vi "New Line from Strings.vi"(0 "Time":string, 1 "Date":string, 2 "Time Stamp":string, 5 "RunName":string, 6 "DAQ Potential (milliVolts)":string, 7 "Delimiter Character":string, 8 "DAQ Resistance (Ohms)":string, 9 "Mode":string, 10 "DAQ Temperature (deg Celsius)":string, 11 "Setting":string, 12 "BK V":string, 13 "BK C":string, 14 "BK R":string, 15 "BK W":string) -> (4 "Line Produced":string)   [LabVIEW 2010]
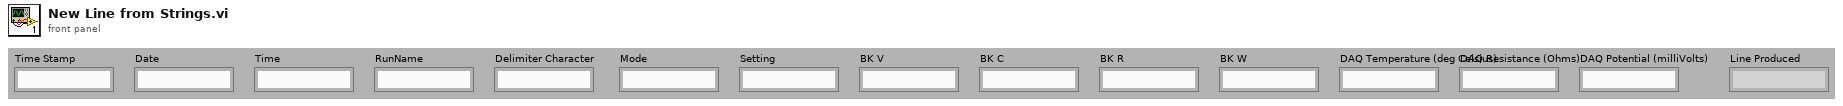
[diagram p1: front panel]
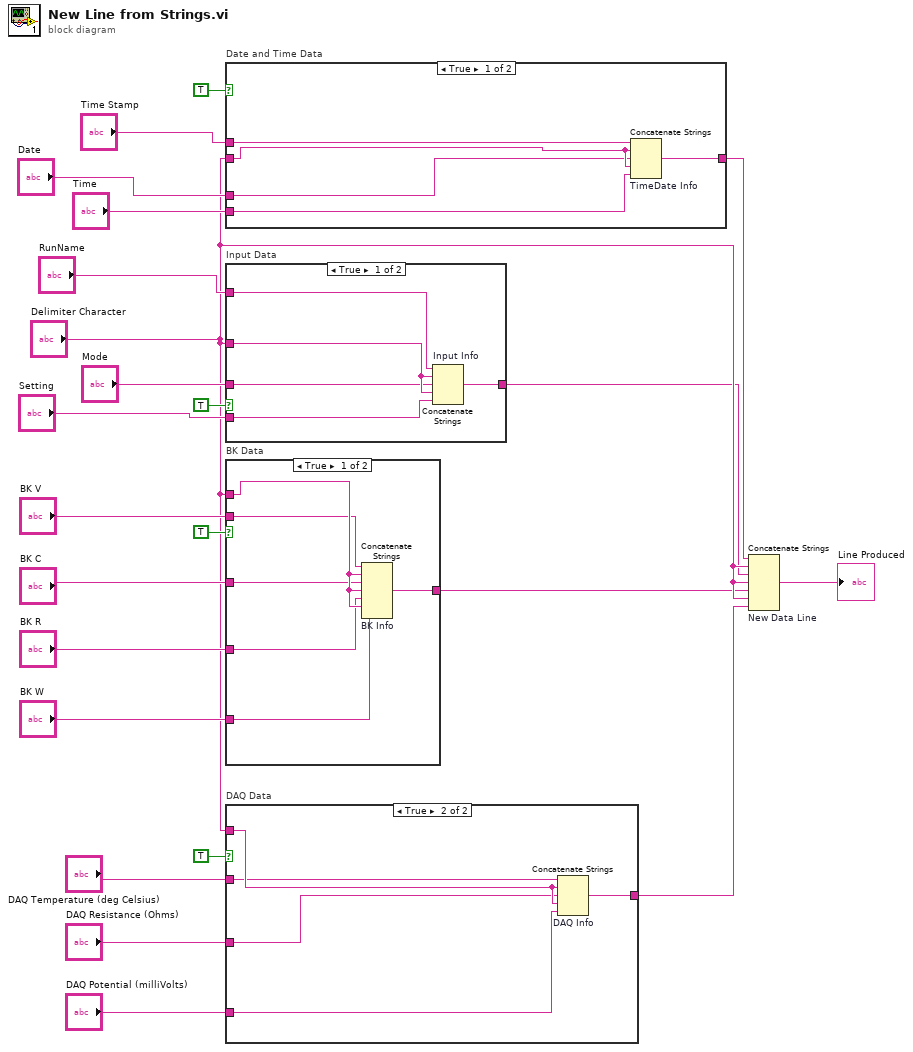
[diagram p0: block diagram]
diagram:
  n1 = case "Date and Time Data" shown="True" TRUE {
    tunnel: "Delimiter Character" -> [w28 w29]
    tunnel: [w27 w29] -> w2
    tunnel: "Time Stamp" -> [w26 _]
    tunnel: "Date" -> [w25 _]
    tunnel: "Time" -> [w24 _]
    frame True {
      n2 = Concatenate Strings "TimeDate Info"(w26, w28, w25, w28, w24) -> (w27:string)
    }
    frame False {
    }
  }
  n3 = case "Input Data" shown="True" TRUE {
    tunnel: "Delimiter Character" -> [w34 w35]
    tunnel: [w33 w35] -> w3
    tunnel: "Setting" -> [w32 _]
    tunnel: "RunName" -> [w31 _]
    tunnel: "Mode" -> [w30 _]
    frame True {
      n4 = Concatenate Strings "Input Info"(w31, w34, w30, w34, w32) -> (w33:string)
    }
    frame False {
    }
  }
  n5 = case "BK Data" shown="True" TRUE {
    tunnel: "Delimiter Character" -> [w40 w42]
    tunnel: [w41 w42] -> w4
    tunnel: "BK V" -> [w39 _]
    tunnel: "BK C" -> [w38 _]
    tunnel: "BK R" -> [w37 _]
    tunnel: "BK W" -> [w36 _]
    frame True {
      n6 = Concatenate Strings "BK Info"(w39, w40, w38, w40, w37, w40, w36) -> (w41:string)
    }
    frame False {
    }
  }
  n7 = case "DAQ Data" shown="True" TRUE {
    tunnel: "Delimiter Character" -> [w43 w48]
    tunnel: [w43 w47] -> w5
    tunnel: "DAQ Temperature (deg Celsius)" -> [_ w46]
    tunnel: "DAQ Resistance (Ohms)" -> [_ w45]
    tunnel: "DAQ Potential (milliVolts)" -> [_ w44]
    frame False {
    }
    frame True {
      n8 = Concatenate Strings "DAQ Info"(w46, w48, w45, w48, w44) -> (w47:string)
    }
  }
  n9 = Concatenate Strings "New Data Line"(w2, "Delimiter Character", w3, "Delimiter Character", w4, "Delimiter Character", w5) -> (→"Line Produced":string)
